vi "PCO_Record.vi"(11 "Hardware.Cameras.PCO":T1) -> ()   [LabVIEW 2014]
panel:
  in  "Exposure (ms)":u32=20
  in  "Exit":bool
  out "Live Preview":u16[][](graph)
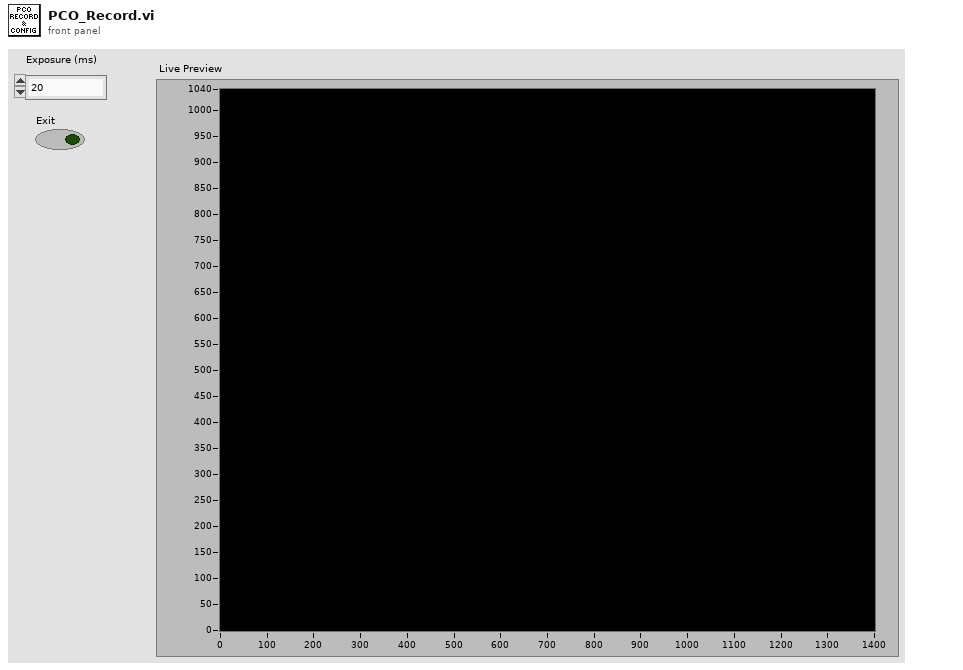
[diagram p1: front panel]
types:
  T1 = cluster{"handle":u64, "BufferID":i16[], "PixelRates":u32[], "Bits/pixel":u16, "SizeHor":u16, "SizeVer":u16}
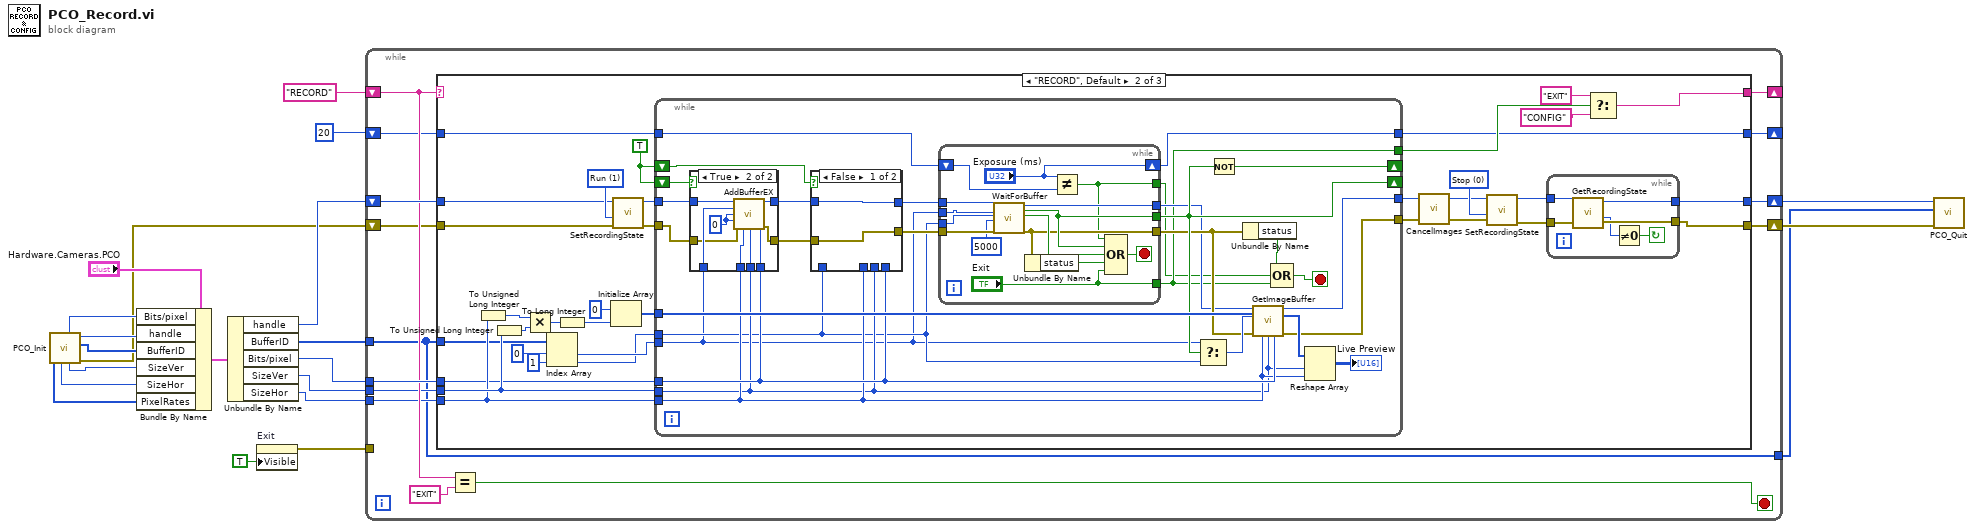
[diagram p0: block diagram]
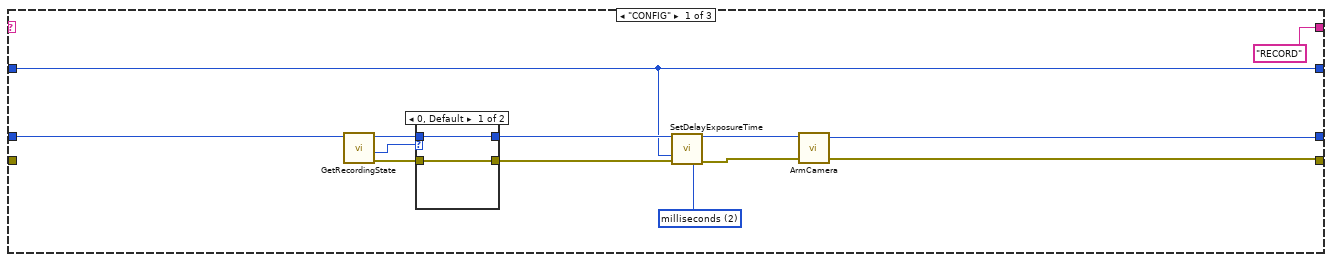
[diagram p2: hidden frame]
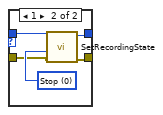
[diagram p3: hidden frame]
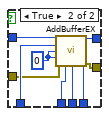
[diagram p5: hidden frame]
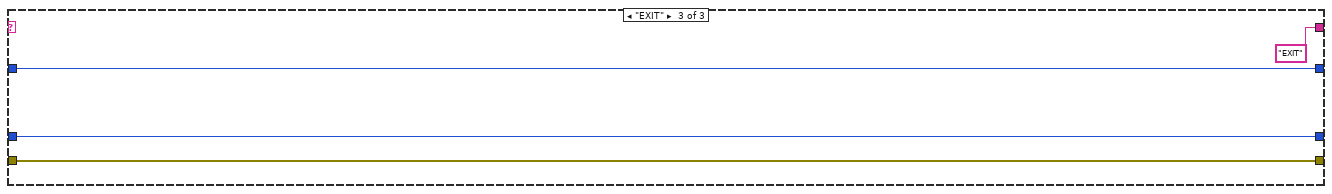
[diagram p6: hidden frame]
diagram:
  n1 = call "PCO_Init.vi"() -> ("ErrorOut"=w2:errorcluster, "BufferID"=w9:i16[], "hout"=w10:u64, "SizeVer"=w8:u16, "Bits/pixel"=w6:u16, "SizeHor"=w7:u16, "PixelRates"=w5:u32[])  [unwired: 5 in]
  n2 = Bundle By Name(cluster="Hardware.Cameras.PCO", "Bits/pixel"=w6, "handle"=w10, "BufferID"=w9, "SizeVer"=w8, "SizeHor"=w7, "PixelRates"=w5) -> (w11:T1)
  n3 = Unbundle By Name(w11) -> ("handle"=w15:u64, "BufferID"=w21:i16[], "Bits/pixel"=w16:u16, "SizeVer"=w17:u16, "SizeHor"=w18:u16)
  n4 = property on="Exit" class="Bool (strict)"("Visible"=TRUE) -> (error out=w13:errorcluster)  [unwired: 2 in, 1 out]
  n5 = while {
    tunnel: w16 -> [w34]
    tunnel: w21 -> [w22]
    shift-right: [w33] -> w4
    shift-left: w15 -> [w35]
    shift-right: [w32] -> _
    shift-left: "RECORD" -> [w31]
    shift-right: [w27] -> _
    shift-left: u32 20 ("Exposure") -> [w28]
    tunnel: w17 -> [w26]
    tunnel: w18 -> [w25]
    tunnel: w13 -> [_]
    shift-right: [w24] -> w3
    shift-left: w2 -> [w23]
    tunnel: [w22] -> w1
    stop <- w29 stop-if-true
    n6 = case shown="\"RECORD\", Default" w31 {
      tunnel: w35 -> [w43 w69 w165]
      tunnel: w26 -> [_ w68 _]
      tunnel: w25 -> [_ w67 _]
      tunnel: w34 -> [_ w66 _]
      tunnel: w22 -> [_ w65 _]
      tunnel: [w42 w64 w165] -> w33
      tunnel: ["RECORD" w61 "EXIT"] -> w32
      tunnel: w28 -> [w37 w59 w164]
      tunnel: [w37 w58 w164] -> w27
      tunnel: [w36 w57 w163] -> w24
      tunnel: w23 -> [_ w56 w163]
      frame "CONFIG" {
        w41 = u16 2 items=["nanoseconds", "microseconds", "milliseconds"] ("ExposureTimeBase")
        n7 = call "GetRecordingState.vi"("ph"=w43) -> ("ErrorOut"=w44:errorcluster, "RecordingState"=w46:u16, "hout"=w45:u64)  [unwired: 3 in, 1 out]
        n8 = case shown="0, Default" w46 {
          tunnel: w45 -> [w50 w54]
          tunnel: w44 -> [w49 w53]
          tunnel: [w50 w52] -> w39
          tunnel: [w49 w51] -> w40
          frame 0, Default {
          }
          frame 1 {
            w55 = u16 0 items=["Stop", "Run"] ("RecordingState")
            n9 = call "SetRecordingState.vi"("ErrorIn"=w53, "RecordingState"=w55, "ph"=w54) -> ("ErrorOut"=w51:errorcluster, "hout"=w52:u64)  [unwired: 2 in, 1 out]
          }
        }
        n10 = call "SetDelayExposureTime.vi"("ph"=w39, "Exposure"=w37, "error in (no error)"=w40, "ExposureTimeBase"=w41) -> ("hout"=w47:u64, "error out"=w48:errorcluster)  [unwired: 9 in, 1 out]
        n11 = call "ArmCamera.vi"("error in (no error)"=w48, "ph"=w47) -> ("error out"=w36:errorcluster, "hout"=w42:u64)  [unwired: 1 in, 1 out]
      }
      frame "RECORD", Default {
        w77 = TRUE
        w87 = u16 1 items=["Stop", "Run"] ("RecordingState")
        w90 = u16 0 items=["Stop", "Run"] ("RecordingState")
        n12 = To Unsigned Long Integer(number=w67) -> (unsigned 32bit integer=w81:u32)
        n13 = To Unsigned Long Integer(number=w68) -> (unsigned 32bit integer=w82:u32)
        n14 = Multiply(x=w81, y=w82) -> (x*y=w74:u32)
        n15 = Index Array(array=w65, index #1=0 ("index"), index #2=1 ("index")) -> (element #1=w72:i16, element #2=w71:i16)
        n16 = To Long Integer(number=w74) -> (32bit integer=w73:i32)
        n17 = Initialize Array(u16 0 ("element"), w73) -> (w83:u16[])
        n18 = call "SetRecordingState.vi"("ErrorIn"=w56, "RecordingState"=w87, "ph"=w69) -> ("ErrorOut"=w86:errorcluster, "hout"=w85:u64)  [unwired: 2 in, 1 out]
        n19 = while {
          tunnel: w72 -> [w95]
          tunnel: w83 -> [w116]
          tunnel: w85 -> [w96]
          tunnel: w68 -> [w101]
          tunnel: w67 -> [w102]
          tunnel: w86 -> [w114]
          tunnel: [w117] -> w78
          tunnel: [w118] -> w70
          tunnel: w71 -> [w99]
          tunnel: w66 -> [w107]
          shift-right: [w105] -> _
          shift-left: w77 -> [w106]
          shift-right: [w103] -> _
          shift-left: w77 -> [w104]
          tunnel: [w94] -> w60
          tunnel: w59 -> [w93]
          tunnel: [w91] -> w58
          stop <- w108 stop-if-true
          n20 = case shown="True" w106 {
            tunnel: [w121 w130] -> w113
            tunnel: [w120 w129] -> w115
            tunnel: w95 -> [_ w128]
            tunnel: w96 -> [w120 w127]
            tunnel: w107 -> [_ w125]
            tunnel: w102 -> [_ w124]
            tunnel: w101 -> [_ w123]
            tunnel: w114 -> [w121 w122]
            frame False {
            }
            frame True {
              w126 = i16 0
              n21 = call "AddBufferEX.vi"("ph"=w127, "BuffNr"=w128, "1stImage"=w126, "LastImage"=w126, "error in (no error)"=w122, "XRes"=w124, "YRes"=w123, "BitPerPixel"=w125) -> ("hout"=w129:u64, "error out"=w130:errorcluster)  [unwired: 5 in, 1 out]
            }
          }
          n22 = case shown="False" w104 {
            tunnel: [w131 w141] -> w109
            tunnel: [w132 w140] -> w110
            tunnel: w99 -> [_ w139]
            tunnel: w115 -> [w132 w138]
            tunnel: w107 -> [_ w136]
            tunnel: w102 -> [_ w135]
            tunnel: w101 -> [_ w134]
            tunnel: w113 -> [w131 w133]
            frame False {
            }
            frame True {
              w137 = i16 0
              n23 = call "AddBufferEX.vi"("ph"=w138, "BuffNr"=w139, "1stImage"=w137, "LastImage"=w137, "error in (no error)"=w133, "XRes"=w135, "YRes"=w134, "BitPerPixel"=w136) -> ("hout"=w140:u64, "error out"=w141:errorcluster)  [unwired: 5 in, 1 out]
            }
          }
          n24 = while {
            tunnel: w95 -> [w153]
            tunnel: w99 -> [w152]
            tunnel: w110 -> [w155]
            tunnel: w109 -> [w154]
            tunnel: [w151] -> w97
            tunnel: [w147] -> w98
            tunnel: [w150] -> w105
            tunnel: ["Exit"] -> w94
            tunnel: [w144] -> w92
            shift-right: ["Exposure (ms)"] -> w91
            shift-left: w93 -> [w145]
            stop <- w156 stop-if-true
            n25 = call "WaitForBuffer.vi"("ph"=w155, "sBufNr"=w153, "sBufNr 2"=w152, "timeout"=5000, "error in (no error)"=w154) -> ("hout"=w151:u64, "Buffer_Ready"=w150:bool, "Buffer_Ready 2"=w149:bool, "error out"=w147:errorcluster)  [unwired: 10 in, 1 out]
            n26 = Unbundle By Name(w147) -> ("status"=w146:bool)
            n27 = Not Equal?(x="Exposure (ms)", y=w145) -> (x != y?=w144:bool)
            n28 = Compound Arithmetic op=OR(w144, w150, w149, w146, "Exit") -> (w156:bool)
          }
          n29 = Select(t=w95, s=w105, f=w99) -> (s? t:f=w112:i16)
          n30 = Not(x=w105) -> (.not. x?=w103:bool)
          n31 = Unbundle By Name(w98) -> ("status"=w100:bool)
          n32 = call "GetImageBuffer.vi"("ph"=w97, "BuffIn"=w116, "BuffNr"=w112, "error in (no error)"=w98, "xRes"=w102, "yRes"=w101, "Bitresolution"=w107) -> ("hout"=w117:u64, "BuffOut"=w119:u16[], "error out"=w118:errorcluster)  [unwired: 5 in, 1 out]
          n33 = Compound Arithmetic op=OR(w100, w92, w94) -> (w108:bool)
          n34 = Reshape Array(w119, w101, w102) -> (→"Live Preview":u16[][])
        }
        n35 = call "CancelImages.vi"("error in (no error)"=w70, "ph"=w78) -> ("error out"=w80:errorcluster, "hout"=w79:u64)  [unwired: 1 in, 1 out]
        n36 = call "SetRecordingState.vi"("ErrorIn"=w80, "RecordingState"=w90, "ph"=w79) -> ("ErrorOut"=w88:errorcluster, "hout"=w89:u64)  [unwired: 2 in, 1 out]
        n37 = while {
          tunnel: [w160] -> w57
          tunnel: w88 -> [w161]
          tunnel: w89 -> [w162]
          tunnel: [w157] -> w64
          stop <- w158 continue-if-true
          n38 = call "GetRecordingState.vi"("ErrorIn"=w161, "ph"=w162) -> ("ErrorOut"=w160:errorcluster, "RecordingState"=w159:u16, "hout"=w157:u64)  [unwired: 2 in, 1 out]
          n39 = Not Equal To 0?(x=w159) -> (x != 0?=w158:bool)
        }
        n40 = Select(t="EXIT", s=w60, f="CONFIG") -> (s? t:f=w61:string)
      }
      frame "EXIT" {
      }
    }
    n41 = Equal?(x=w31, y="EXIT") -> (x = y?=w29:bool)
  }
  n42 = call "PCO_Quit.vi"("error in"=w3, "Array"=w1, "ph"=w4) -> ()  [unwired: 8 in, 1 out]
